vi "updateJumperPositionsBasedOnNewStageZero.vi"(8 "error in":errorcluster, 9 "preZeroStageCooridinates":i32[](array[numeric]), 11 "JumperPositions":T1) -> (0 "error out":errorcluster)   [LabVIEW 2015]
panel:
  # "Stage:"
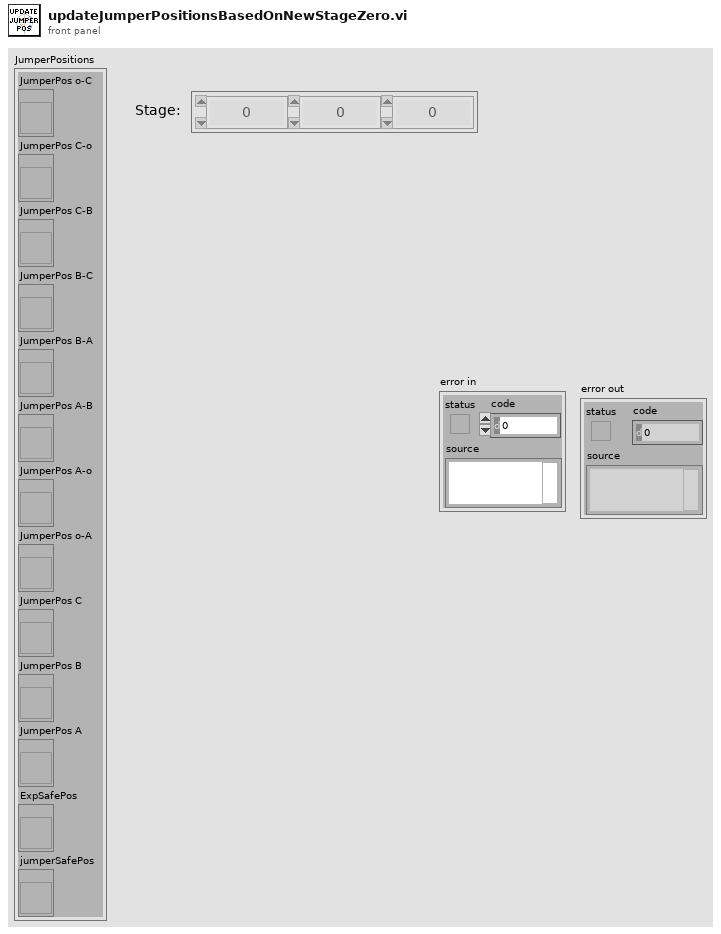
[diagram p1: front panel]
types:
  T1 = cluster{"JumperPos o-C":refnum<vi>, "JumperPos C-o":refnum<vi>, "JumperPos C-B":refnum<vi>, "JumperPos B-C":refnum<vi>, "JumperPos B-A":refnum<vi>, "JumperPos A-B":refnum<vi>, "JumperPos A-o":refnum<vi>, "JumperPos o-A":refnum<vi>, "JumperPos C":refnum<vi>, "JumperPos B":refnum<vi>, "JumperPos A":refnum<vi>, "ExpSafePos":refnum<vi>, "jumperSafePos":refnum<vi>}
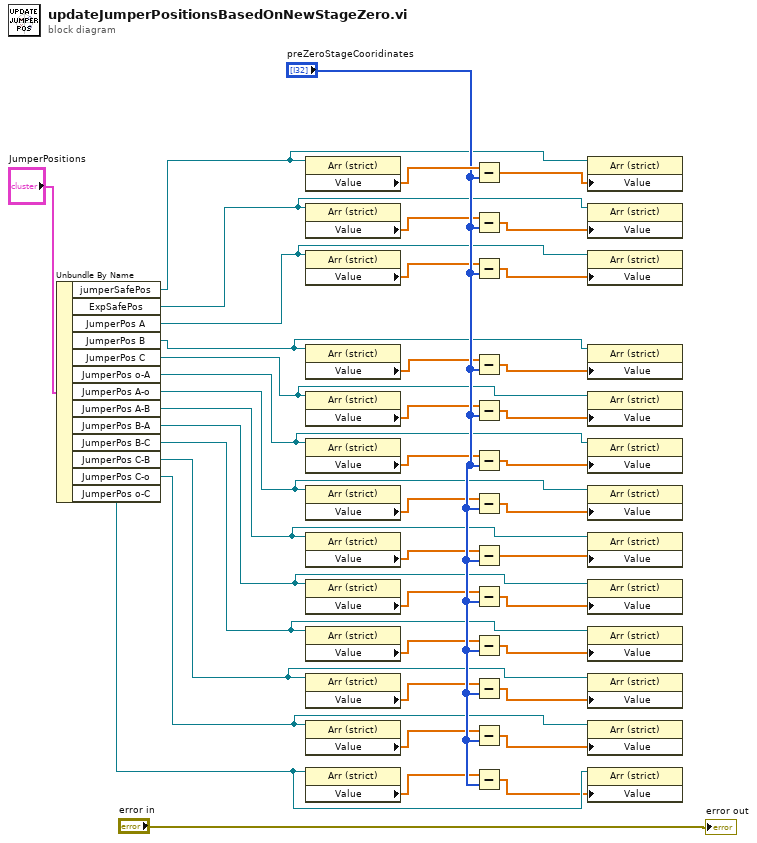
[diagram p0: block diagram]
diagram:
  n1 = Unbundle By Name("JumperPositions") -> ("jumperSafePos"=w36:refnum<vi>, "ExpSafePos"=w35:refnum<vi>, "JumperPos A"=w34:refnum<vi>, "JumperPos B"=w33:refnum<vi>, "JumperPos C"=w32:refnum<vi>, "JumperPos o-A"=w31:refnum<vi>, "JumperPos A-o"=w30:refnum<vi>, "JumperPos A-B"=w29:refnum<vi>, "JumperPos B-A"=w28:refnum<vi>, "JumperPos B-C"=w27:refnum<vi>, "JumperPos C-B"=w26:refnum<vi>, "JumperPos C-o"=w25:refnum<vi>, "JumperPos o-C"=w24:refnum<vi>)
  n2 = property class="Arr (strict)"(reference=w36) -> ("Value"=w41:dbl[])  [unwired: 1 in, 2 out]
  n3 = property class="Arr (strict)"(reference=w35) -> ("Value"=w38:dbl[])  [unwired: 1 in, 2 out]
  n4 = property class="Arr (strict)"(reference=w34) -> ("Value"=w22:dbl[])  [unwired: 1 in, 2 out]
  n5 = property class="Arr (strict)"(reference=w33) -> ("Value"=w23:dbl[])  [unwired: 1 in, 2 out]
  n6 = property class="Arr (strict)"(reference=w32) -> ("Value"=w19:dbl[])  [unwired: 1 in, 2 out]
  n7 = property class="Arr (strict)"(reference=w31) -> ("Value"=w17:dbl[])  [unwired: 1 in, 2 out]
  n8 = property class="Arr (strict)"(reference=w30) -> ("Value"=w15:dbl[])  [unwired: 1 in, 2 out]
  n9 = property class="Arr (strict)"(reference=w29) -> ("Value"=w13:dbl[])  [unwired: 1 in, 2 out]
  n10 = property class="Arr (strict)"(reference=w28) -> ("Value"=w11:dbl[])  [unwired: 1 in, 2 out]
  n11 = property class="Arr (strict)"(reference=w27) -> ("Value"=w9:dbl[])  [unwired: 1 in, 2 out]
  n12 = property class="Arr (strict)"(reference=w26) -> ("Value"=w7:dbl[])  [unwired: 1 in, 2 out]
  n13 = property class="Arr (strict)"(reference=w25) -> ("Value"=w5:dbl[])  [unwired: 1 in, 2 out]
  n14 = property class="Arr (strict)"(reference=w24) -> ("Value"=w3:dbl[])  [unwired: 1 in, 2 out]
  n15 = Subtract(x=w41, y="preZeroStageCooridinates") -> (x-y=w40:dbl[])
  n16 = Subtract(x=w38, y="preZeroStageCooridinates") -> (x-y=w37:dbl[])
  n17 = Subtract(x=w22, y="preZeroStageCooridinates") -> (x-y=w21:dbl[])
  n18 = Subtract(x=w23, y="preZeroStageCooridinates") -> (x-y=w20:dbl[])
  n19 = Subtract(x=w19, y="preZeroStageCooridinates") -> (x-y=w18:dbl[])
  n20 = Subtract(x=w17, y="preZeroStageCooridinates") -> (x-y=w16:dbl[])
  n21 = Subtract(x=w15, y="preZeroStageCooridinates") -> (x-y=w14:dbl[])
  n22 = Subtract(x=w13, y="preZeroStageCooridinates") -> (x-y=w12:dbl[])
  n23 = Subtract(x=w11, y="preZeroStageCooridinates") -> (x-y=w10:dbl[])
  n24 = Subtract(x=w9, y="preZeroStageCooridinates") -> (x-y=w8:dbl[])
  n25 = Subtract(x=w7, y="preZeroStageCooridinates") -> (x-y=w6:dbl[])
  n26 = Subtract(x=w5, y="preZeroStageCooridinates") -> (x-y=w4:dbl[])
  n27 = Subtract(x=w3, y="preZeroStageCooridinates") -> (x-y=w2:dbl[])
  n28 = property class="Arr (strict)"(reference=w36, "Value"=w40) -> ()  [unwired: 1 in, 2 out]
  n29 = property class="Arr (strict)"(reference=w35, "Value"=w37) -> ()  [unwired: 1 in, 2 out]
  n30 = property class="Arr (strict)"(reference=w34, "Value"=w21) -> ()  [unwired: 1 in, 2 out]
  n31 = property class="Arr (strict)"(reference=w33, "Value"=w20) -> ()  [unwired: 1 in, 2 out]
  n32 = property class="Arr (strict)"(reference=w32, "Value"=w18) -> ()  [unwired: 1 in, 2 out]
  n33 = property class="Arr (strict)"(reference=w31, "Value"=w16) -> ()  [unwired: 1 in, 2 out]
  n34 = property class="Arr (strict)"(reference=w30, "Value"=w14) -> ()  [unwired: 1 in, 2 out]
  n35 = property class="Arr (strict)"(reference=w29, "Value"=w12) -> ()  [unwired: 1 in, 2 out]
  n36 = property class="Arr (strict)"(reference=w28, "Value"=w10) -> ()  [unwired: 1 in, 2 out]
  n37 = property class="Arr (strict)"(reference=w27, "Value"=w8) -> ()  [unwired: 1 in, 2 out]
  n38 = property class="Arr (strict)"(reference=w26, "Value"=w6) -> ()  [unwired: 1 in, 2 out]
  n39 = property class="Arr (strict)"(reference=w25, "Value"=w4) -> ()  [unwired: 1 in, 2 out]
  n40 = property class="Arr (strict)"(reference=w24, "Value"=w2) -> ()  [unwired: 1 in, 2 out]
  "error out" <- "error in"
